vi "Register Logger.vi"(8 "error in (no error)":errorcluster, 9 "Task ID":string, 10 "EnQr":refnum<class "Message Enqueuer.lvclass">, 11 "LoggingManager in":refnum<class "LoggingManager.lvclass">) -> (0 "error out":errorcluster, 3 "LoggingManager out":refnum<class "LoggingManager.lvclass">)   [LabVIEW 2020, in "VolatusDataLogger.lvlib" / "LoggingManager.lvclass"]
uses:
  LoggingManager.lvclass
  C:/dev/lv20CE/relink/lv-volatus/Volatus/Task/Task.lvclass
  <vilib>/ActorFramework/Message Enqueuer/Message Enqueuer.lvclass
  LoggingManager.lvclass/LoggingManager.ctl
  Volatus/Task/Task.lvclass/Task.ctl
  Volatus/Event API/EventAPI.lvclass/EventAPI.ctl
  Volatus/EventHandler Messages/Handle Event Msg/Handle Event Msg.lvclass/Handle Event Msg.ctl
  <vilib>/ActorFramework/Message Enqueuer/Message Enqueuer.lvclass/Message Enqueuer.ctl
  Volatus/EventHandler Messages/Handle Event Msg/Send Handle Event.vi
  <vilib>/ActorFramework/Message Enqueuer/Enqueue.vi
  Volatus/EventHandler Messages/Handle Event Msg/Handle Event Msg.lvclass
  C:/Program Files (x86)/National Instruments/LabVIEW 2020/vi.lib/ActorFramework/Message/Message.lvclass
  Volatus/Task/Task ID.vi
  <vilib>/ActorFramework/Message Priority Queue/Priority Enqueue.vi
  Volatus/Task/Task.lvclass
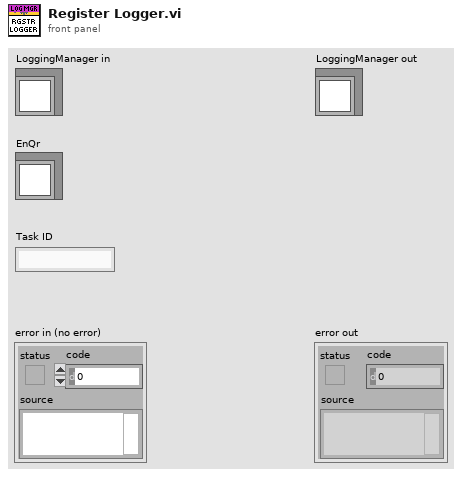
[diagram p1: front panel]
types:
  T1 = map{string, refnum<class "Message Enqueuer.lvclass">}
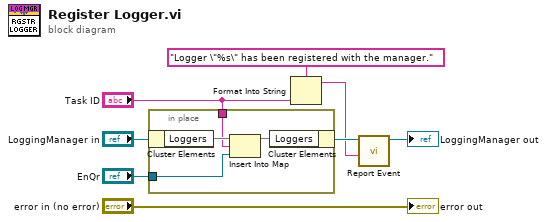
[diagram p0: block diagram]
diagram:
  n1 = in-place {
    in-place-border: "Task ID" -> [w11]
    in-place-border: "EnQr" -> [w10]
    n2 = in-place-cluster #1("LoggingManager in") -> ("Loggers"=w12:T1)
    n3 = Insert Into Map(map in=w12, key=w11, value=w10) -> (map out=w9:T1)  [unwired: 2 out]
    n4 = in-place-cluster #1("Loggers"=w9) -> (w5:refnum<class "LoggingManager.lvclass">)
  }
  n5 = Format Into String(format string="Logger \"%s\" has been registered with the manager.", "Task ID") -> (resulting string=w1:string)  [unwired: 2 in, 1 out]
  n6 = call "Report Event.vi"("Message"=w1, "Task in"=w5) -> ("Task out"=→"LoggingManager out":refnum<class "LoggingManager.lvclass">)  [unwired: 8 in, 1 out]
  "error out" <- "error in (no error)"
